vi "TWM Client Test.vi"() -> ()   [LabVIEW 2020, in "TWM Client.lvlib"]
uses:
  TWM Client.lvlib
  TWM Client Result Max Dim.ctl
  TWM Client Quantity Record.ctl
panel:
  out "data":T1[][](array[typedef])
  in  "qwtb maxdim (scalar)":T2 caption="Max. shown dimension (scalar)"
  in  "quantity names (all)":string[](array[string])
  in  "meas root path (last)":path
  in  "btn get result":bool
  in  "btn stop":bool
  out "aux message":string
  out "ready?":bool
  in  "btn start":bool
  in  "btn exit":bool
  out "channel idns":string[](array[string])
  in  "btn set meas":bool
  in  "btn idn":bool
  in  "command string":string="#startsection:: Set measurement\n  #startsection:: sampling\n    sample count:: 10000\n    sampling rate [Hz]:: 10000\n    aperture [s]:: 10e-6\n    repetition cycles:: 10\n  #endsection:: sampling\n  #startsection:: processing\n    #startsection:: qwtb\n      algorithm ID:: TWM-FPNLSF\n      #startmatrix:: list of parameter names\n        f_est\n      #endmatrix:: list of parameter names\n      #startmatrix:: f_est\n        400\n      #endmatrix:: f_est\n    #endsection:: qwtb\n  #endsection:: processing\n#endsection:: Set measurement"
  out "error out":errorcluster
  in  "pipe name":string="\\\\.\\pipe\\TWM:server" caption="Named Pipe Identifier"
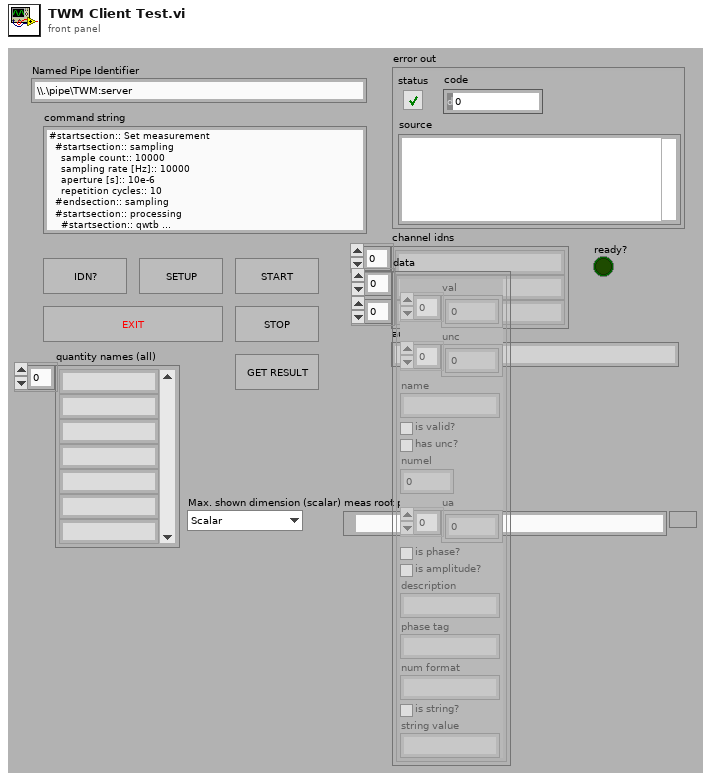
[diagram p1: front panel]
types:
  T1 = typedef "TWM Client.lvlib/TWM Client Quantity Record.ctl" = cluster{"val":dbl[], "unc":dbl[], "name":string, "is valid?":bool, "has unc?":bool, "numel":i32, "ua":dbl[], "is phase?":bool, "is amplitude?":bool, "description":string, "phase tag":string, "num format":string, "is string?":bool, "string value":string}
  T2 = typedef "TWM Client.lvlib/TWM Client Result Max Dim.ctl" = enum16{"Scalar", "Vector", "Matrix"}
  T3 = enum16{"CREATE_NEW", "CREATE_ALWAYS", "OPEN_EXISTING", "OPEN_ALWAYS", "TRUNCATE_EXISTING"}
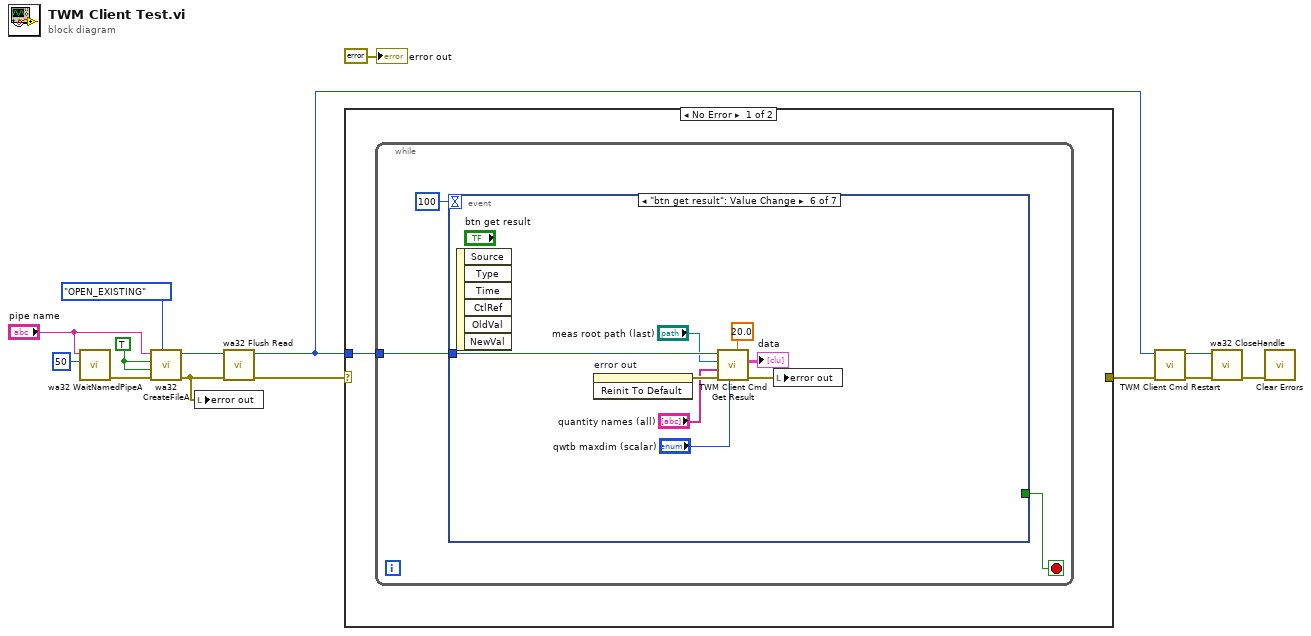
[diagram p0: block diagram]
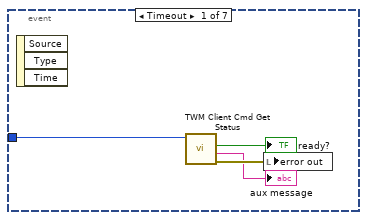
[diagram p2: hidden frame]
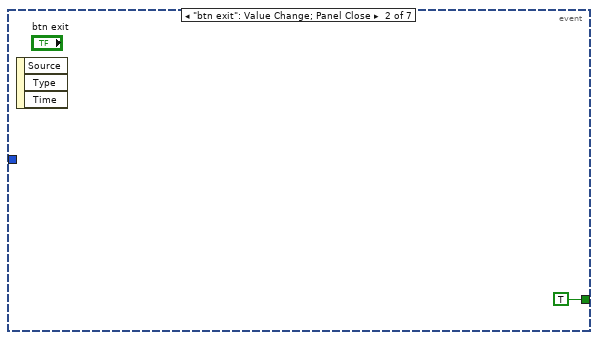
[diagram p3: hidden frame]
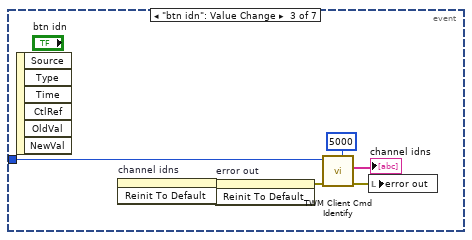
[diagram p4: hidden frame]
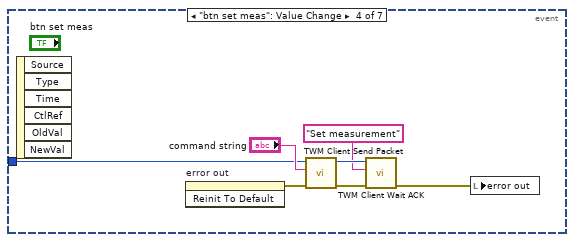
[diagram p5: hidden frame]
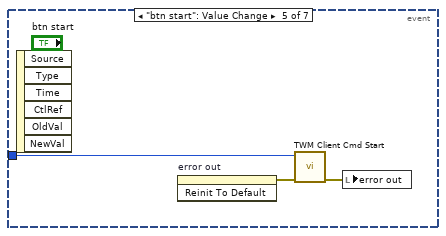
[diagram p6: hidden frame]
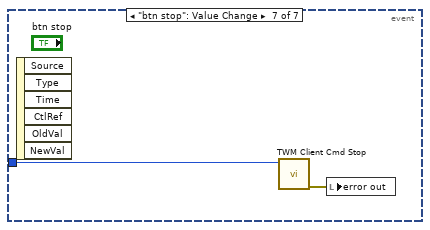
[diagram p7: hidden frame]
diagram:
  w14 = TRUE ("read")
  n1 = call "wa32 WaitNamedPipeA.vi"("timeout [ms]"=u32 50, "pipe name"="pipe name") -> ("error out"=w12:errorcluster)  [unwired: 9 in]
  n2 = call "wa32 CreateFileA.vi"("creation dispozition"=T3."OPEN_EXISTING", "error in"=w12, "write"=w14, "read"=w14, "file path"="pipe name") -> ("error out"=w4:errorcluster, "handle"=w1:i32)  [unwired: 5 in]
  n3 = local write "error out"(w4) -> ()
  n4 = call "wa32 Flush Read.vi"("error in"=w4, "handle"=w1) -> ("error out"=w3:errorcluster, "handle out"=w2:i32)  [unwired: 7 in, 1 out]
  n5 = case shown="No Error" w3 {
    selector: w3 -> [_ w50]
    tunnel: [_ w50] -> w7
    tunnel: w2 -> [w15 _]
    frame No Error {
      n6 = while {
        tunnel: w15 -> [w18]
        stop <- w17 stop-if-true
        n7 = event shown="[5] \"btn get result\": Value Change" {
          selector: _ -> [_ _ _ _ _ _ _]
          dyn-events: _ -> [_ _ _ _ _ _ _]
          timeout: 100 -> [_ _ _ _ _ _ _]
          tunnel: w18 -> [w22 _ w25 w34 w37 w45 w49]
          tunnel: [_ TRUE _ _ _ _ _] -> w17
          event Timeout {
            n8 = event-data() -> ()  [unwired: 1 in, 3 out]
            n9 = call "TWM Client Cmd Get Status.vi"("handle"=w22) -> ("error out"=w21:errorcluster, "error message"=→"aux message":string, "ready?"=→"ready?":bool)  [unwired: 6 in, 2 out]
            n10 = local write "error out"(w21) -> ()
          }
          event "btn exit": Value Change; Panel Close {
            n11 = event-data() -> ()  [unwired: 1 in, 3 out]
          }
          event "btn idn": Value Change {
            n12 = event-data() -> ()  [unwired: 1 in, 6 out]
            n13 = invoke on="channel idns" class="Arr (strict)" method="Reinit To Default"() -> (error out=w27:errorcluster)  [unwired: 3 in, 2 out]
            n14 = invoke on="error out" class="Clust (strict)" method="Reinit To Default"(error in=w27) -> (error out=w26:errorcluster)  [unwired: 2 in, 2 out]
            n15 = call "TWM Client Cmd Identify.vi"("timeout [ms]"=5000, "error in"=w26, "handle"=w25) -> ("error out"=w29:errorcluster, "channel idns"=→"channel idns":string[])  [unwired: 5 in, 2 out]
            n16 = local write "error out"(w29) -> ()
          }
          event "btn set meas": Value Change {
            n17 = event-data() -> ()  [unwired: 1 in, 6 out]
            n18 = invoke on="error out" class="Clust (strict)" method="Reinit To Default"() -> (error out=w35:errorcluster)  [unwired: 3 in, 2 out]
            n19 = call "TWM Client Send Packet.vi"("error in"=w35, "command string"="command string", "handle"=w34) -> ("error out"=w33:errorcluster, "handle out"=w32:i32)  [unwired: 7 in]
            n20 = call "TWM Client Wait ACK.vi"("error in"=w33, "command header"="Set measurement" ("key string"), "handle"=w32) -> ("error out"=w31:errorcluster)  [unwired: 7 in, 1 out]
            n21 = local write "error out"(w31) -> ()
          }
          event "btn start": Value Change {
            n22 = event-data() -> ()  [unwired: 1 in, 6 out]
            n23 = invoke on="error out" class="Clust (strict)" method="Reinit To Default"() -> (error out=w39:errorcluster)  [unwired: 3 in, 2 out]
            n24 = call "TWM Client Cmd Start.vi"("error in"=w39, "handle"=w37) -> ("error out"=w38:errorcluster)  [unwired: 8 in, 1 out]
            n25 = local write "error out"(w38) -> ()
          }
          event "btn get result": Value Change {
            n26 = event-data() -> ()  [unwired: 1 in, 6 out]
            n27 = invoke on="error out" class="Clust (strict)" method="Reinit To Default"() -> (error out=w47:errorcluster)  [unwired: 3 in, 2 out]
            n28 = call "TWM Client Cmd Get Result.vi"("timeout [s] (10s)"=20.0, "qwtb maxdim (scalar)"="qwtb maxdim (scalar)", "error in"=w47, "quantity names (all)"="quantity names (all)", "meas root path (last)"="meas root path (last)", "handle"=w45) -> ("error out"=w46:errorcluster, "result data"=→"data":T1[][])  [unwired: 2 in, 2 out]
            n29 = local write "error out"(w46) -> ()
          }
          event "btn stop": Value Change {
            n30 = event-data() -> ()  [unwired: 1 in, 6 out]
            n31 = call "TWM Client Cmd Stop.vi"("handle"=w49) -> ("error out"=w48:errorcluster)  [unwired: 9 in, 1 out]
            n32 = local write "error out"(w48) -> ()
          }
        }
      }
    }
    frame Error {
    }
  }
  n33 = call "TWM Client Cmd Restart.vi"("error in"=w7, "handle"=w2) -> ("error out"=w6:errorcluster, "handle out"=w5:i32)  [unwired: 8 in]
  n34 = call "wa32 CloseHandle.vi"("error in"=w6, "handle"=w5) -> ("error out"=w9:errorcluster)  [unwired: 9 in]
  n35 = call <vilib>:"Clear Errors.vi"("error in (no error)"=w9) -> ()  [unwired: 5 in, 2 out]
  "error out" <- errorcluster {"status"=FALSE, "code"=0, "source"=""} ("error out")
